vi "initialise.vi"(8 "error in (no error)":errorcluster, 11 "DL090430TriggeredExperimentController in":refnum<class "ExperimentControllerDL090430DAQmxTriggered.lvclass">) -> (0 "error out":errorcluster, 3 "DL090430TriggeredExperimentController out":refnum<class "ExperimentControllerDL090430DAQmxTriggered.lvclass">)   [LabVIEW 2010, in "ExperimentControllerDL090430DAQmxTriggered.lvclass"]
uses:
  ExperimentControllerDL090430DAQmxTriggered.lvclass
  GenericExperimentController/GenericExperimentController/GenericExperimentController.lvclass
  ExperimentControllerDL090430DAQmxTriggered.lvclass/ExperimentControllerDL090430DAQmxTriggered.ctl
  <vilib>/DAQmx/create/channels.llb/DAQmx Create Channel (AI-Voltage-Basic).vi
  <vilib>/DAQmx/configure/timing.llb/DAQmx Timing (Sample Clock).vi
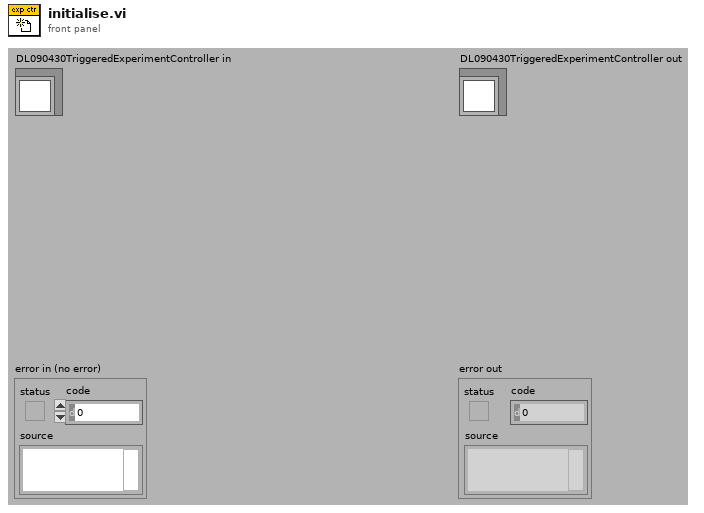
[diagram p1: front panel]
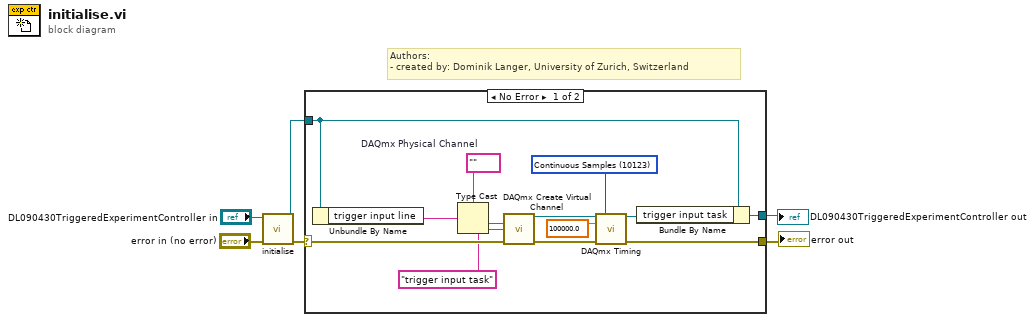
[diagram p0: block diagram]
diagram:
  # "Authors: \n- created by: Dominik Langer, University of Zurich, Switzerland"
  n1 = call-parent "initialise.vi"("error in (no error)"="error in (no error)", "GenericPlugin in"="DL090430TriggeredExperimentController in") -> ("error out"=w4:errorcluster, "GenericPlugin out"=w3:refnum<class "ExperimentControllerDL090430DAQmxTriggered.lvclass">)  [unwired: 8 out]
  n2 = case shown="No Error" w4 {
    selector: w4 -> [w17 w20]
    tunnel: w3 -> [w19 w21]
    tunnel: [w7 w20] -> w2
    tunnel: [w18 w21] -> w1
    frame No Error {
      w9 = 10123 items=["Finite Samples"=10178, "Continuous Samples"=10123, "Hardware Timed Single Point"=12522] ("sample mode")
      w15 = tag ""  # DAQmx Physical Channel
      n3 = Unbundle By Name(w19) -> ("trigger input line"=w13:string)
      n4 = Type Cast(type=w15, x=w13) -> (*(type *) &x=w14:tag)
      n5 = call-poly <vilib>:"DAQmx Create Virtual Channel.vi"("physical channels"=w14, "name to assign"="trigger input task", "error in"=w17) -> ("task out"=w11:refnum<k21>, "error out"=w12:errorcluster)  [unwired: 6 in, 5 out]
      n6 = call-poly <vilib>:"DAQmx Timing.vi"("task/channels in"=w11, "sample mode"=w9, "rate"=100000.0, "error in"=w12) -> ("task out"=w8:refnum<k21>, "error out"=w7:errorcluster)  [unwired: 3 in, 7 out]
      n7 = Bundle By Name(cluster=w19, "trigger input task"=w8) -> (w18:refnum<class "ExperimentControllerDL090430DAQmxTriggered.lvclass">)
    }
    frame Error {
    }
  }
  "error out" <- w2
  "DL090430TriggeredExperimentController out" <- w1
